vi "cam-vision.vi"(8 "error in":errorcluster, 11 "main-national data in":T1) -> (0 "error out":errorcluster, 2 "Array":string[][](array[string]), 3 "main-national data out":T1)   [LabVIEW 2019]
uses:
  ctl/main data-national.ctl
  ctl/position set.ctl
panel:
  out "Image Buffer":T3(plugin-control)
  out "Image Out":T3(plugin-control)
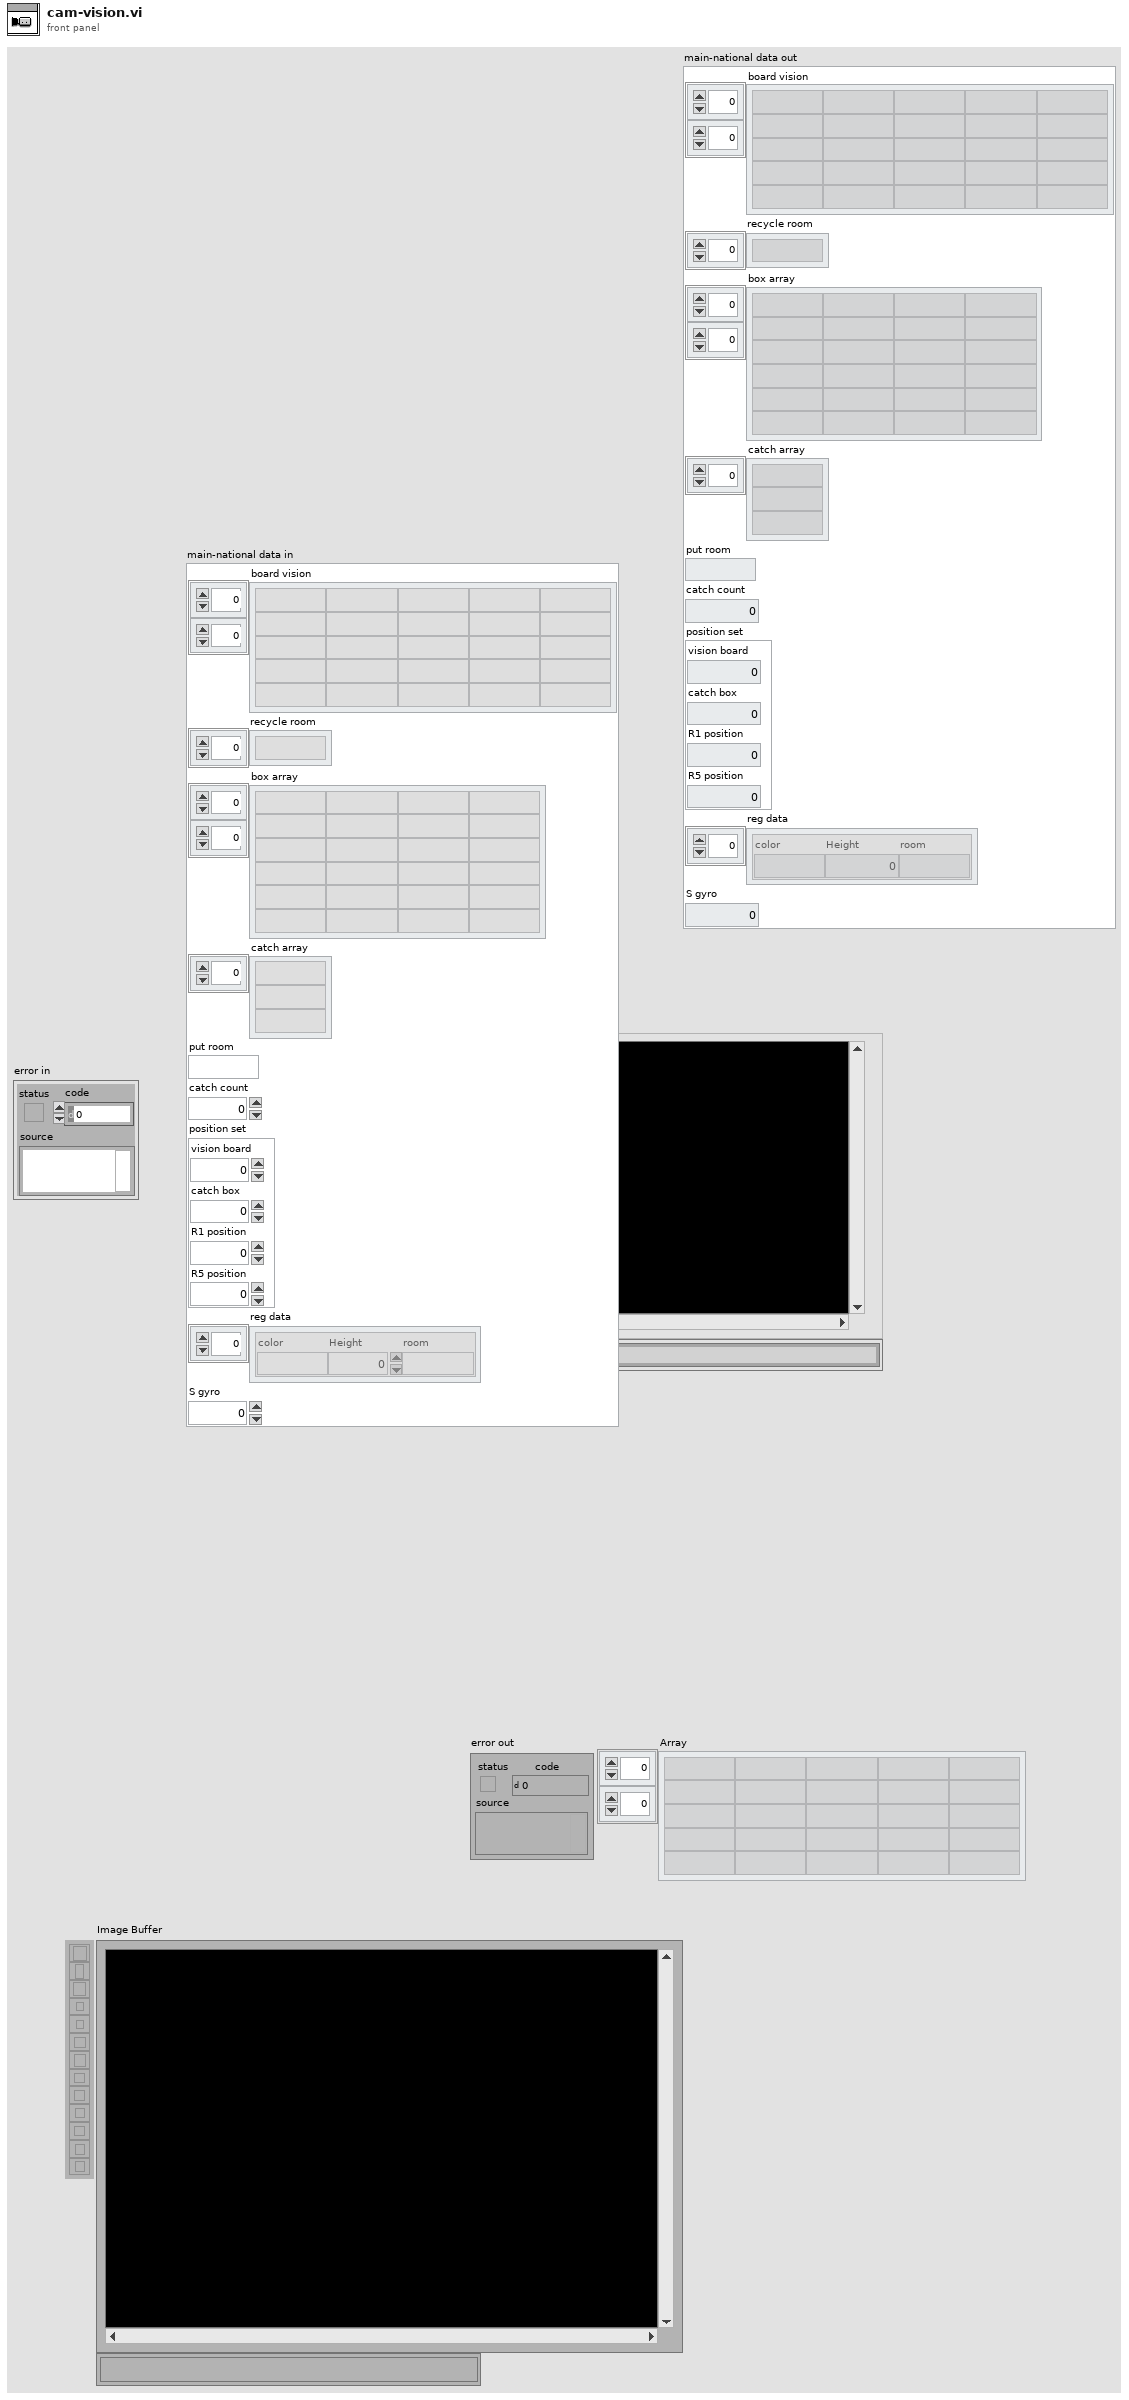
[diagram p1: front panel]
types:
  T1 = typedef "main data-national.ctl" = cluster{"board vision":string[][], "recycle room":string[], "box array":string[][], "catch array":string[], "put room":string, "catch count":dbl, "position set":T2, "reg data":cluster{"color":string, "Height":i32, "room":string}[], "S gyro":dbl}
  T2 = typedef "position set.ctl" = cluster{"vision board":dbl, "catch box":dbl, "R1 position":dbl, "R5 position":dbl}
  T3 = typedef "IMAQ Image.ctl" = refnum<image>
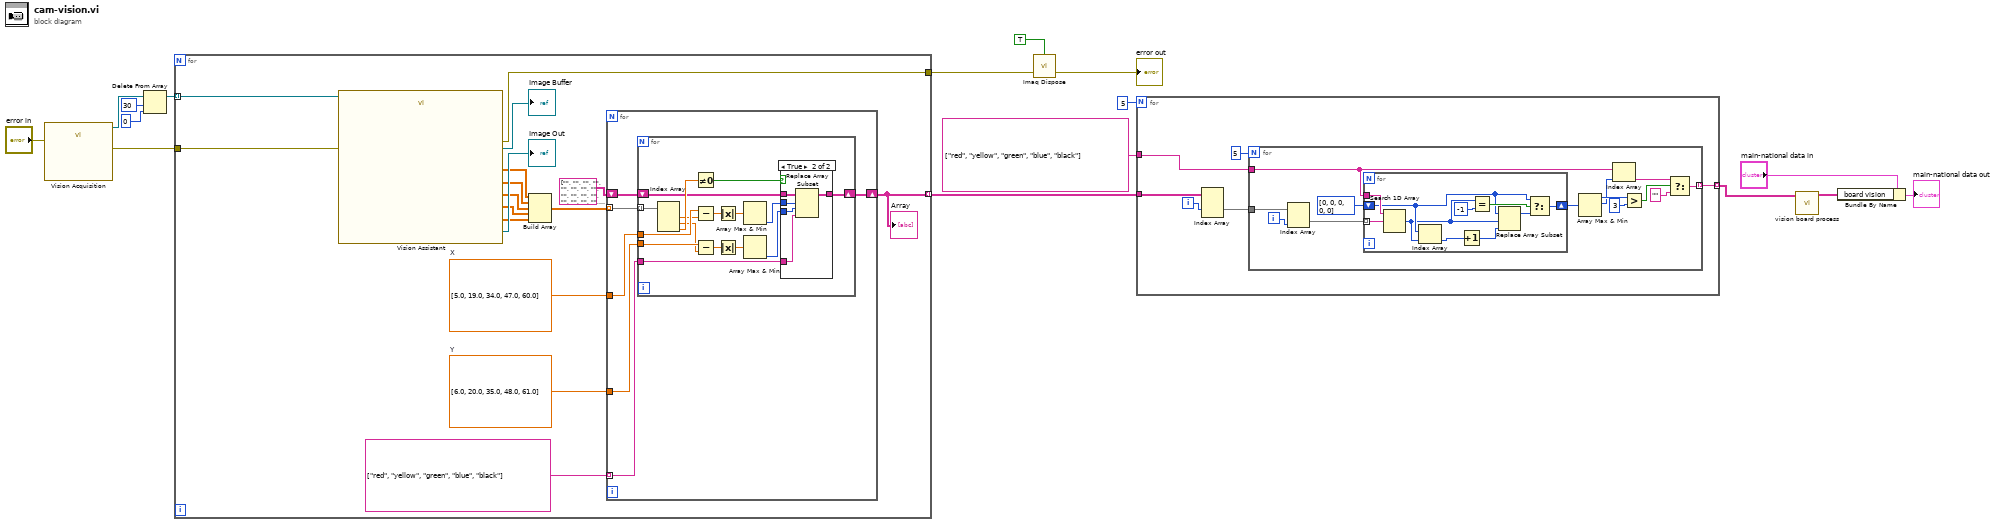
[diagram p0: block diagram]
diagram:
  n1 = call "Vision Acquisition"("error in"="error in") -> ("All Images Out"=w9:T3[], "error out"=w10:errorcluster)  [unwired: 25 in]
  n2 = Delete From Array(array=w9, length=30, index=0) -> (array with subset deleted=w5:T3[])  [unwired: 1 out]
  n3 = for {
    tunnel: [w26] -> w16
    tunnel: [w19] -> w6 mode=indexing
    tunnel: w10 -> [w18]
    tunnel: w5 -> [w17] mode=indexing
    w21 = dbl[] [6.0, 20.0, 35.0, 48.0, 61.0]  # Y
    w22 = dbl[] [5.0, 19.0, 34.0, 47.0, 60.0]  # X
    n4 = call "Vision Assistant"("Image In"=w17, "error in"=w18) -> ("Image Buffer (Image Buffer 5)"=→"Image Buffer":T3, "Particle Measurements (Pixels) (red)"=w31:dbl[][], "Particle Measurements (Pixels) (yellow)"=w30:dbl[][], "Particle Measurements (Pixels) (green)"=w27:dbl[][], "Particle Measurements (Pixels) (blue)"=w28:dbl[][], "Particle Measurements (Pixels) (black)"=w29:dbl[][], "Image Buffer (Image Buffer 7)"=→"Image Out":T3, "error out"=w26:errorcluster)  [unwired: 17 in, 1 out]
    n5 = Build Array(w31, w30, w27, w28, w29) -> (w24:dbl[][][])
    n6 = for {
      tunnel: string[] ["red", "yellow", "green", "blue", "black"] -> [w37] mode=indexing
      tunnel: w24 -> [w38] mode=indexing
      tunnel: w22 -> [w36]
      tunnel: w21 -> [w35]
      shift-right: [w33] -> w19
      shift-left: string[][] [["", "", "", "", ""], ["", "", "", "", ""], ["", "", "", "", ""], ["", "", "", "", ""], ["", "", "", "", ""]] -> [w34]
      n7 = for {
        tunnel: w38 -> [w54] mode=indexing
        tunnel: w37 -> [w40]
        tunnel: w36 -> [w51]
        tunnel: w35 -> [w49]
        shift-right: [w39] -> w33
        shift-left: w34 -> [w43]
        n8 = Index Array(array=w54) -> (element #1=w50:dbl, element #2=w48:dbl, element #3=w52:dbl)  [unwired: 3 in]
        n9 = Not Equal To 0?(x=w52) -> (x != 0?=w53:bool)
        n10 = Subtract(x=w51, y=w50) -> (x-y=w47:dbl[])
        n11 = Subtract(x=w49, y=w48) -> (x-y=w46:dbl[])
        n12 = Absolute Value(x=w47) -> (abs(x)=w44:dbl[])
        n13 = Absolute Value(x=w46) -> (abs(x)=w45:dbl[])
        n14 = Array Max & Min(array=w44) -> (min index (indices)=w42:i32)  [unwired: 3 out]
        n15 = Array Max & Min(array=w45) -> (min index (indices)=w41:i32)  [unwired: 3 out]
        n16 = case shown="True" w53 {
          tunnel: w43 -> [w55 w60]
          tunnel: w42 -> [_ w59]
          tunnel: w41 -> [_ w58]
          tunnel: w40 -> [_ w57]
          tunnel: [w55 w56] -> w39
          frame False {
          }
          frame True {
            n17 = Replace Array Subset(array=w60, new element=w57, index (row)=w59, index (col)=w58) -> (w56:string[][])
          }
        }
      }
    }
    "Array" <- w19
  }
  n18 = call "Imaq Dispose"("All Images? (No)"=TRUE, "error in (no error)"=w16) -> ("error out"=→"error out":errorcluster)  [unwired: 4 in]
  n19 = for {
    N: 5 -> [_]
    tunnel: w6 -> [w65]
    tunnel: string[] ["red", "yellow", "green", "blue", "black"] -> [w63]
    tunnel: [w62] -> w2 mode=indexing
    i -> [w61]
    n20 = Index Array(array=w65, index (dim 1)=w61) -> (element=w64:string[][])  [unwired: 2 in]
    n21 = for {
      N: 5 -> [_]
      tunnel: w64 -> [w79]
      tunnel: w63 -> [w72]
      tunnel: [w69] -> w62 mode=indexing
      i -> [w67]
      n22 = Index Array(array=w79, index (col)=w67) -> (element=w78:string[])  [unwired: 1 in]
      n23 = for {
        tunnel: w78 -> [w88] mode=indexing
        tunnel: w72 -> [w89]
        shift-right: [w80] -> w76
        shift-left: i32[] [0, 0, 0, 0, 0] -> [w84]
        n24 = Search 1D Array(1D array=w89, element=w88) -> (index of element=w82:i32)  [unwired: 1 in]
        n25 = Index Array(array=w84, index=w82) -> (element=w85:i32)
        n26 = Increment(x=w85) -> (x+1=w83:i32)
        n27 = Equal?(x=w82, y=-1) -> (x = y?=w86:bool)
        n28 = Replace Array Subset(array=w84, new element=w83, index=w82) -> (w81:i32[])
        n29 = Select(t=w84, s=w86, f=w81) -> (s? t:f=w80:i32[])
      }
      n30 = Array Max & Min(array=w76) -> (max value=w71:i32, max index (indices)=w68:i32)  [unwired: 2 out]
      n31 = Index Array(array=w72, index=w68) -> (element=w70:string)
      n32 = Greater?(x=w71, y=3) -> (0:w74:bool)
      n33 = Select(t=w70, s=w74, f="") -> (s? t:f=w69:string)
    }
  }
  n34 = call "vision board process.vi"("Array in"=w2) -> ("Array out"=w1:string[][])  [unwired: 10 in]
  n35 = Bundle By Name(cluster="main-national data in", "board vision"=w1) -> (→"main-national data out":T1)
